vi "PreMatch LCD.vi"(6 "Communication Value:":dbl, 7 "Autonomous Mode":bool, 8 "error in":errorcluster, 9 "Camera":dbl, 10 "Distance":dbl, 11 "PSI":dbl) -> (0 "error out":errorcluster)   [LabVIEW 2013]
panel:
  out "Result String 2:":string
  out "Result String 1:":string
  # "0: no camera communication\n1: Camera Communication, not hot goal\n2: Camera Communication, hot goal"
  # "1Ball"
  # "0"
  # "1"
  # "2 Ball"
  # "0-999"
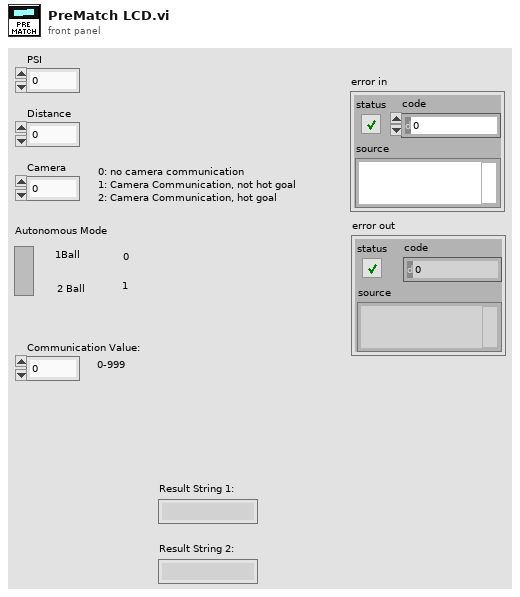
[diagram p1: front panel]
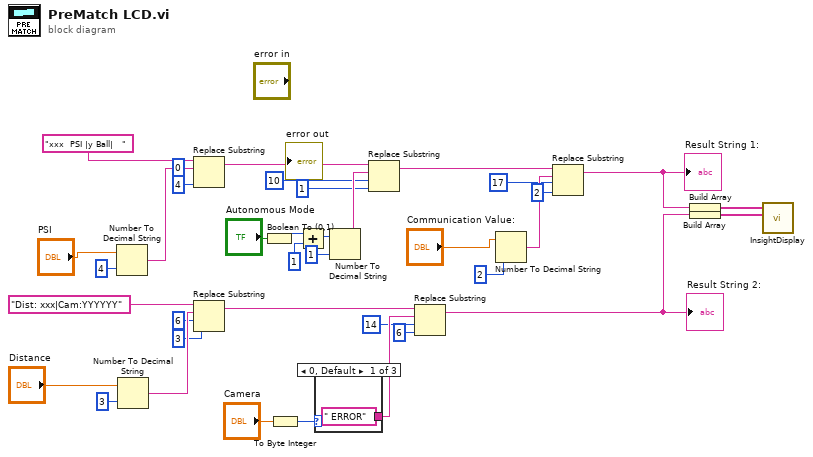
[diagram p0: block diagram]
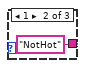
[diagram p2: hidden frame]
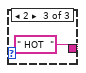
[diagram p3: hidden frame]
diagram:
  n1 = Number To Decimal String(number="PSI", width (-)=i16 4) -> (decimal integer string=w34:string)
  n2 = Number To Decimal String(number="Distance", width (-)=i16 3) -> (decimal integer string=w12:string)
  n3 = Replace Substring(2:4 ("length (len. of substring)"), 3:0 ("offset (0)"), 4:w34, 5:"xxx  PSI |y Ball|   ") -> (1:w31:string)  [unwired: 1 out]
  n4 = Replace Substring(2:3 ("length (len. of substring)"), 3:6 ("offset (0)"), 4:w12, 5:"Dist: xxx|Cam:YYYYYY") -> (1:w6:string)  [unwired: 1 out]
  n5 = Boolean To (0,1)(Boolean="Autonomous Mode") -> (0, 1=w29:i16)
  n6 = To Byte Integer(number="Camera") -> (8bit integer=w8:i8)
  n7 = Add(x=w29, y=i16 1) -> (x+y=w2:i16)
  n8 = case shown="0, Default" w8 {
    tunnel: [" ERROR" "NotHot" " HOT  "] -> w7
    frame 0, Default {
    }
    frame 1 {
    }
    frame 2 {
    }
  }
  n9 = Number To Decimal String(number=w2, width (-)=i16 1) -> (decimal integer string=w27:string)
  n10 = Replace Substring(2:1 ("length (len. of substring)"), 3:10 ("offset (0)"), 4:w27, 5:w31) -> (1:w19:string)  [unwired: 1 out]
  n11 = Replace Substring(2:6 ("length (len. of substring)"), 3:14 ("offset (0)"), 4:w7, 5:w6) -> (1:w5:string)  [unwired: 1 out]
  "Result String 2:" <- w5
  n12 = Number To Decimal String(number="Communication Value:", width (-)=i16 2) -> (decimal integer string=w24:string)
  n13 = Replace Substring(2:2 ("length (len. of substring)"), 3:17 ("offset (0)"), 4:w24, 5:w19) -> (1:w18:string)  [unwired: 1 out]
  "Result String 1:" <- w18
  n14 = Build Array(w18) -> (w17:string[])
  n15 = Build Array(w5) -> (w16:string[])
  n16 = call "InsightDisplay.vi"("Zone 2 Data"=w16, "Zone 1 Data"=w17) -> ()  [unwired: 10 in]
